vi "Timestamp Offset.vi"(11 "Timestamp":timestamp) -> (3 "Timezone offset string":string)   [LabVIEW 2013, in "JKI JSON Serialization.lvlib" / "JSON Serializer.lvclass"]
uses:
  JSON Serializer.lvclass
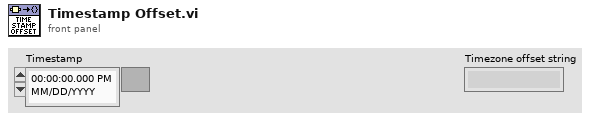
[diagram p1: front panel]
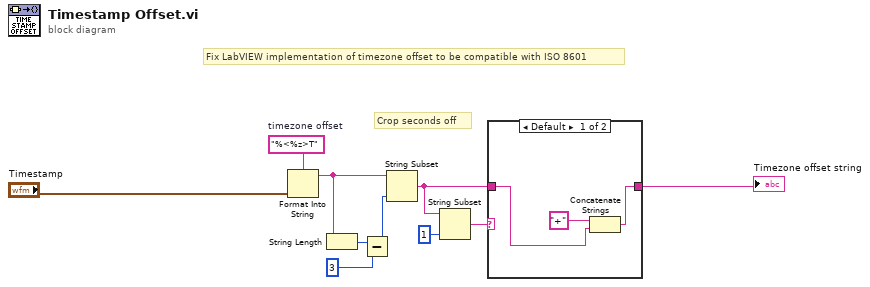
[diagram p0: block diagram]
diagram:
  w8 = "%<%z>T"  # timezone offset
  # "Crop seconds off"
  # "Fix LabVIEW implementation of timezone offset to be compatible with ISO 8601"
  n1 = Format Into String(format string=w8, "Timestamp") -> (resulting string=w7:string)  [unwired: 2 in, 1 out]
  n2 = String Length(string=w7) -> (length=w6:i32)
  n3 = Subtract(x=w6, y=3) -> (x-y=w4:i32)
  n4 = String Subset(string=w7, length (rest)=w4) -> (substring=w1:string)  [unwired: 1 in]
  n5 = String Subset(string=w1, length (rest)=1 ("length (rest)")) -> (substring=w2:string)  [unwired: 1 in]
  n6 = case shown="Default" w2 {
    tunnel: [w13 w14] -> w9
    tunnel: w1 -> [w11 w14]
    frame Default {
      n7 = Concatenate Strings("+", w11) -> (w13:string)
    }
    frame "-" {
    }
  }
  "Timezone offset string" <- w9
